vi "pyclass_test.vi"() -> ()   [LabVIEW 2022 SP3]
panel:
  out "error out":errorcluster
  out "Numeric":dbl
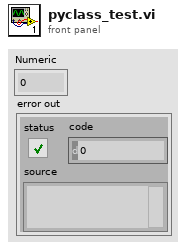
[diagram p1: front panel]
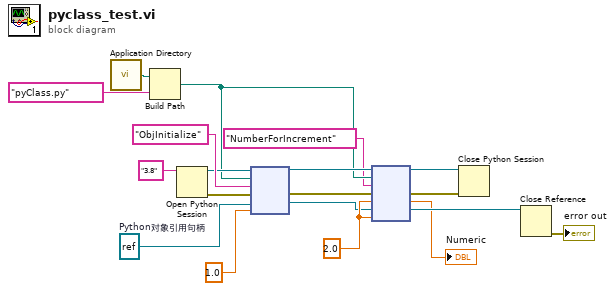
[diagram p0: block diagram]
diagram:
  w7 = 2.0
  w13 = refnum<k38> refnum  # Python对象引用句柄
  n1 = call <vilib>:"Application Directory.vi"() -> ("Application Directory"=w19:path)
  n2 = Build Path(base path=w19, name or relative path="pyClass.py" ("名称或相对路径")) -> (appended path=w10:path)
  n3 = Open Python Session(python version="3.8" ("Python version")) -> (session out=w14:refnum<k35>, error out=w15:errorcluster)  [unwired: 2 in]
  n4 = node(w14, w10, "ObjInitialize" ("函数名称"), w15, w13, 1.0) -> (w11:refnum<k35>, w8:errorcluster, w6:refnum<k38>)  [unwired: 1 in, 2 out]
  n5 = node(w11, w10, "NumberForIncrement" ("函数名称"), w8, w7, w6, w7) -> (w5:refnum<k35>, w4:errorcluster, →"Numeric":dbl, w3:refnum<k38>)  [unwired: 1 in, 2 out]
  n6 = Close Python Session(session in=w5, error in=w4) -> ()  [unwired: 1 out]
  n7 = Close Reference(reference=w3) -> (error out=→"error out":errorcluster)  [unwired: 1 in]
